vi "CUDA GEMM And Operations Float.vi"(11 "dimension size":i32=16384) -> (3 "CUDA Time":dbl)   [LabVIEW 2020]
uses:
  Cuda/Source/Methods/Memory Control/SGL/CreateTensor&HTD(2DArraySGL).vi
  Cuda/Source/Methods/Functions/CuBLAS/SGL/gemm(SGL).vi
  Cuda/Source/Methods/Functions/Numeric/SGL/Add Array Scalar(SGL).vi
  Cuda/Source/Methods/Functions/Array/SGL/Max & Min(SGL).vi
  Cuda/Source/Tensor.lvclass
  <vilib>/Analysis/NI_AALBase.lvlib
panel:
  out "max value":dbl
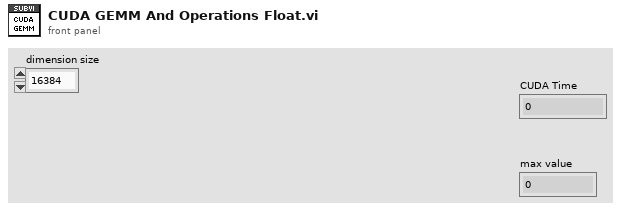
[diagram p1: front panel]
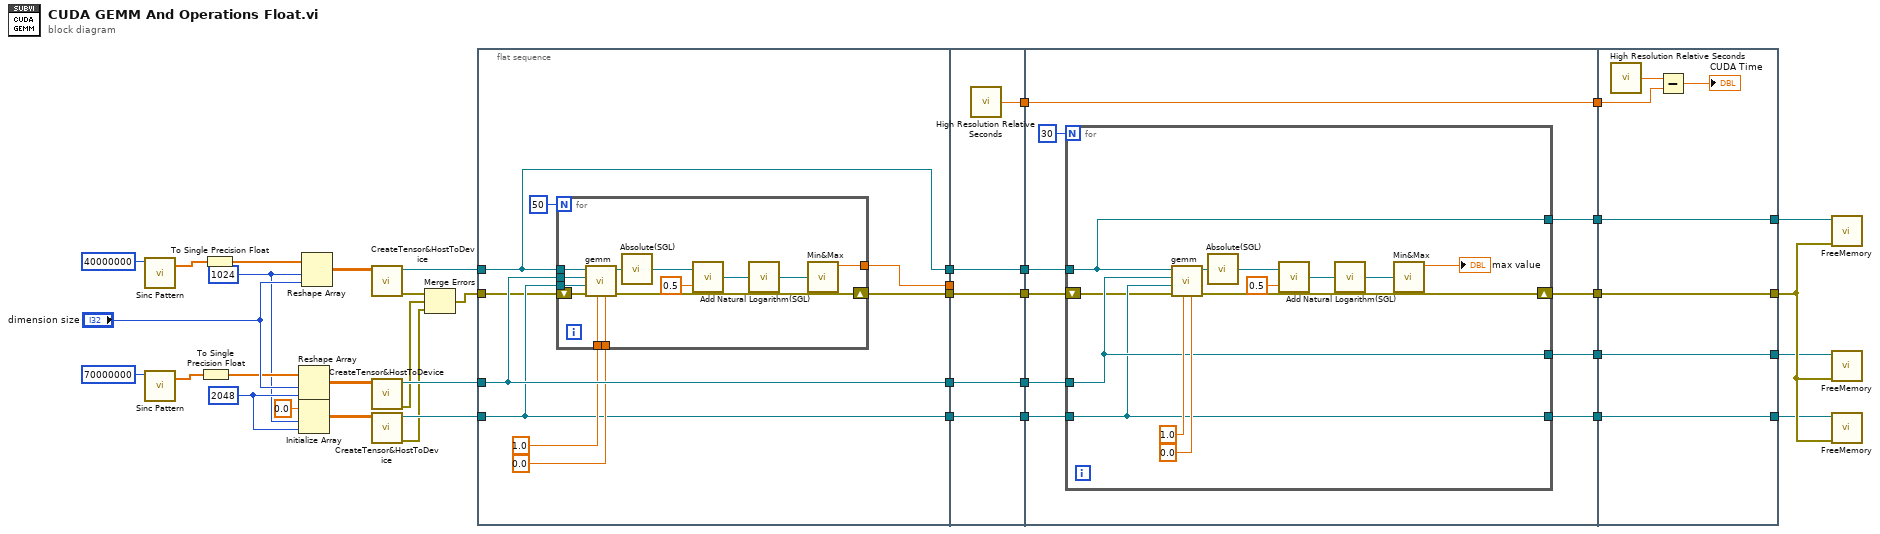
[diagram p0: block diagram]
diagram:
  w17 = 2048 ("dimension size")
  w16 = 1024 ("dimension size")
  n1 = call <vilib>:"Sinc Pattern.vi"("samples"=40000000) -> ("Sinc Pattern"=w31:dbl[])  [unwired: 3 in, 1 out]
  n2 = call <vilib>:"Sinc Pattern.vi"("samples"=70000000) -> ("Sinc Pattern"=w30:dbl[])  [unwired: 3 in, 1 out]
  n3 = To Single Precision Float(number=w30) -> (single precision float=w27:sgl[])
  n4 = To Single Precision Float(number=w31) -> (single precision float=w28:sgl[])
  n5 = Reshape Array(w27, "dimension size", w17) -> (w21:sgl[][])
  n6 = Initialize Array(sgl 0.0 ("element"), w16, w17) -> (w14:sgl[][])
  n7 = Reshape Array(w28, w16, "dimension size") -> (w23:sgl[][])
  n8 = call-poly "CreateTensor&HostToDevice.vi"("data"=w23) -> ("error out"=w4:errorcluster, "Tensor out"=w22:refnum<class "Tensor.lvclass">)  [unwired: 9 in]
  n9 = call-poly "CreateTensor&HostToDevice.vi"("data"=w21) -> ("error out"=w1:errorcluster, "Tensor out"=w20:refnum<class "Tensor.lvclass">)  [unwired: 9 in]
  n10 = call-poly "CreateTensor&HostToDevice.vi"("data"=w14) -> ("error out"=w2:errorcluster, "Tensor out"=w18:refnum<class "Tensor.lvclass">)  [unwired: 9 in]
  n11 = Merge Errors(w4, w1, w2) -> (w3:errorcluster)
  n12 = flat-sequence {
    tunnel: w18 -> [w43]
    tunnel: w20 -> [w47]
    tunnel: w22 -> [w48]
    tunnel: [w47] -> w26
    tunnel: [w43] -> w25
    tunnel: [w48] -> w24
    tunnel: [w44] -> w19
    tunnel: [w41] -> w6
    tunnel: w3 -> [w40]
    tunnel: [w66] -> w39
    tunnel: [w65] -> w38
    tunnel: [w64] -> w37
    tunnel: [w63] -> w36
    tunnel: w26 -> [w64]
    tunnel: w25 -> [w63]
    tunnel: w24 -> [w65]
    tunnel: w19 -> [_]
    tunnel: w6 -> [w62]
    tunnel: [w62] -> w5
    tunnel: w39 -> [w76]
    tunnel: [w76] -> w35
    tunnel: w38 -> [w75]
    tunnel: w37 -> [w74]
    tunnel: w36 -> [w73]
    tunnel: [w72] -> w34
    tunnel: [w70] -> w12
    tunnel: [w69] -> w10
    tunnel: [w68] -> w8
    tunnel: w5 -> [w67]
    tunnel: w35 -> [w95]
    tunnel: w34 -> [w93]
    tunnel: [w93] -> w13
    tunnel: w12 -> [w92]
    tunnel: [w92] -> w11
    tunnel: w10 -> [w91]
    tunnel: [w91] -> w9
    tunnel: w8 -> [w90]
    tunnel: [w90] -> w7
    frame #0 {
      n13 = for {
        N: 50 -> [_]
        tunnel: w48 -> [w61]
        tunnel: w47 -> [w60]
        tunnel: sgl 1.0 ("alpha") -> [w59]
        tunnel: sgl 0.0 ("beta") -> [w58]
        tunnel: [w52] -> w44
        tunnel: w43 -> [w51]
        shift-right: [w50] -> w41
        shift-left: w40 -> [w49]
        n14 = call-poly "gemm.vi"("b"=w58, "a"=w59, "error in"=w49, "C"=w51, "B"=w60, "A"=w61) -> ("error out"=w50:errorcluster, "C"=w57:refnum<class "Tensor.lvclass">)  [unwired: 4 in]
        n15 = call "Absolute(SGL).vi"("x"=w57) -> ("abs(x)"=w56:refnum<class "Tensor.lvclass">)
        n16 = call-poly "Add.vi"("y"=sgl 0.5, "x"=w56) -> ("x + y"=w54:refnum<class "Tensor.lvclass">)
        n17 = call "Natural Logarithm(SGL).vi"("x"=w54) -> ("ln(x)"=w53:refnum<class "Tensor.lvclass">)
        n18 = call-poly "Min&Max.vi"("array"=w53) -> ("max value"=w52:sgl)  [unwired: 4 in, 3 out]
      }
    }
    frame #1 {
      n19 = call <vilib>:"High Resolution Relative Seconds.vi"() -> ("relative seconds"=w66:dbl)
    }
    frame #2 {
      n20 = for {
        N: 30 -> [_]
        tunnel: w75 -> [w80]
        tunnel: w74 -> [w79]
        tunnel: w73 -> [w78]
        tunnel: [w80] -> w70
        tunnel: [w79] -> w69
        tunnel: [w78] -> w68
        shift-right: [w81] -> w72
        shift-left: w67 -> [w77]
        n21 = call-poly "gemm.vi"("b"=0.0 ("beta"), "a"=1.0 ("alpha"), "error in"=w77, "C"=w78, "B"=w79, "A"=w80) -> ("error out"=w81:errorcluster, "C"=w85:refnum<class "Tensor.lvclass">)  [unwired: 4 in]
        n22 = call "Absolute(SGL).vi"("x"=w85) -> ("abs(x)"=w86:refnum<class "Tensor.lvclass">)
        n23 = call-poly "Add.vi"("y"=sgl 0.5, "x"=w86) -> ("x + y"=w88:refnum<class "Tensor.lvclass">)
        n24 = call "Natural Logarithm(SGL).vi"("x"=w88) -> ("ln(x)"=w89:refnum<class "Tensor.lvclass">)
        n25 = call-poly "Min&Max.vi"("array"=w89) -> ("max value"=→"max value":sgl)  [unwired: 4 in, 3 out]
      }
    }
    frame #3 {
      n26 = call <vilib>:"High Resolution Relative Seconds.vi"() -> ("relative seconds"=w96:dbl)
      n27 = Subtract(x=w96, y=w95) -> (x-y=→"CUDA Time":dbl)
    }
  }
  n28 = call "FreeMemory.vi"("error in"=w13, "Tensor in"=w11) -> ()  [unwired: 9 in, 1 out]
  n29 = call "FreeMemory.vi"("error in"=w13, "Tensor in"=w9) -> ()  [unwired: 9 in, 1 out]
  n30 = call "FreeMemory.vi"("error in"=w13, "Tensor in"=w7) -> ()  [unwired: 9 in, 1 out]
